vi "SparaRead.vi"(1 "Test Summary":string) -> (0 "判定结果":bool[](array[boolean]))   [LabVIEW 2011]
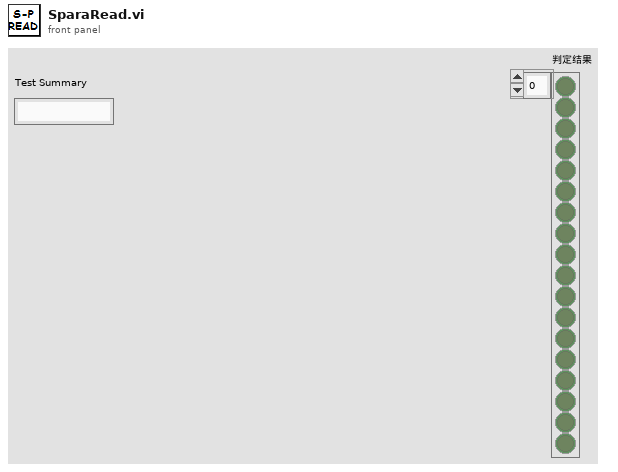
[diagram p1: front panel]
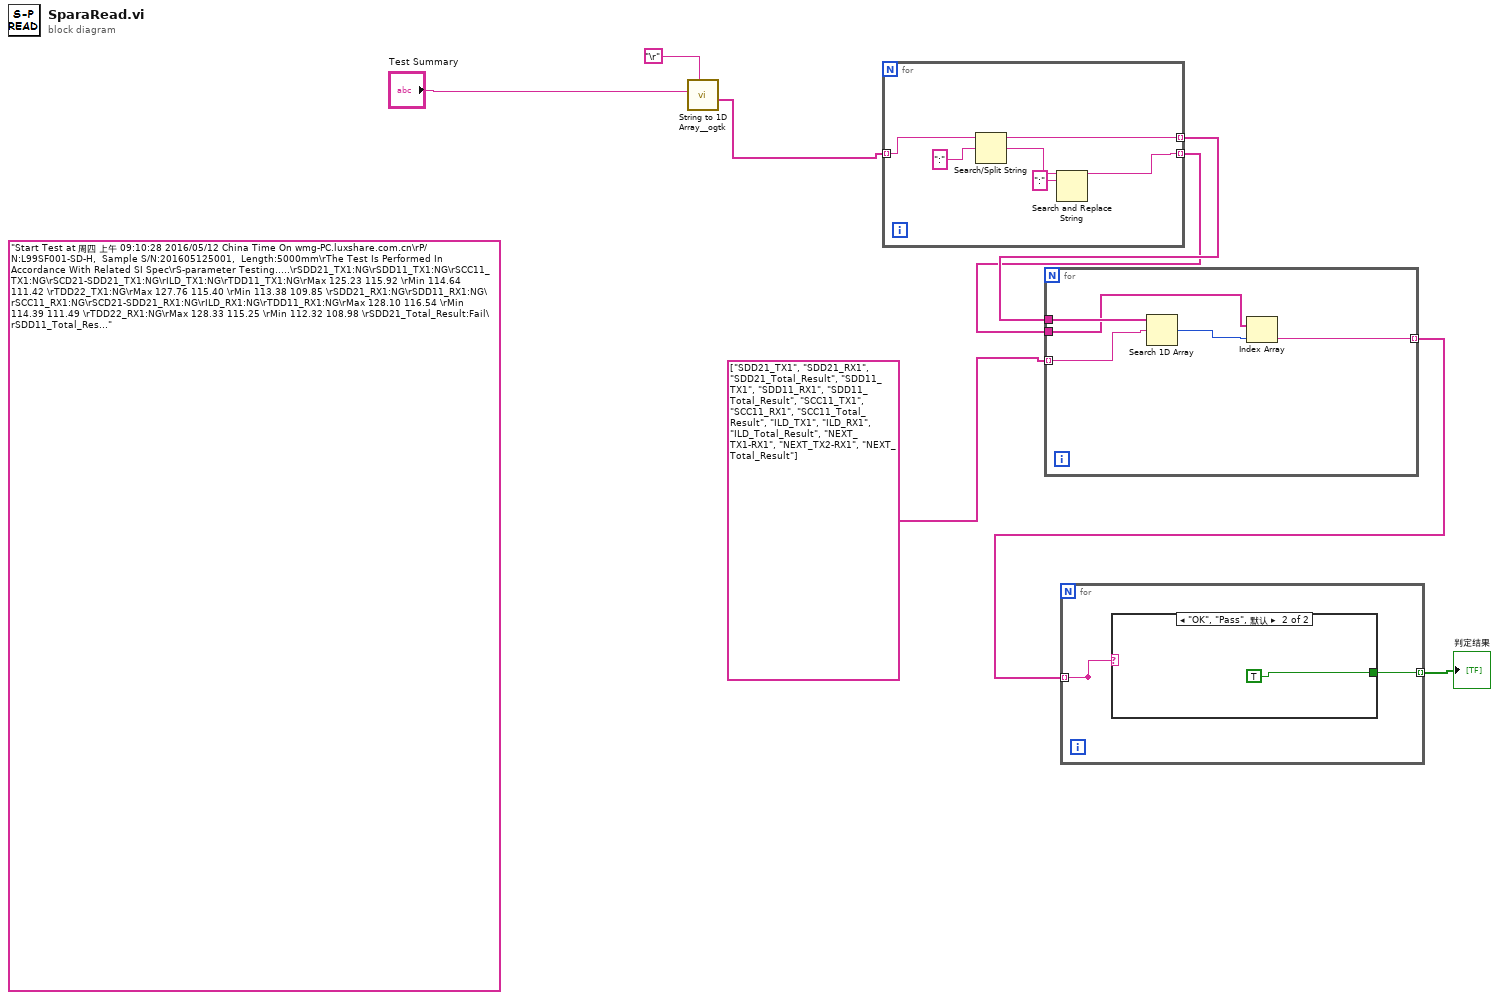
[diagram p0: block diagram]
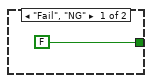
[diagram p2: hidden frame]
diagram:
  (unwired) "Start Test at 周四 上午 09:10:28 2016/05/12 China Time On wmg-PC.luxshare.com.cn\rP/N:L99SF001-SD-H,  Sample S/N:201605125001,  Length:5000mm\rThe Test Is Performed In Accordance With Related SI Spec\rS-parameter Testing.....\rSDD21_TX1:NG\rSDD11_TX1:NG\rSCC11_TX1:NG\rSCD21-SDD21_TX1:NG\rILD_TX1:NG\rTDD11_TX1:NG\rMax 125.23 115.92 \rMin 114.64 111.42 \rTDD22_TX1:NG\rMax 127.76 115.40 \rMin 113.38 109.85 \rSDD21_RX1:NG\rSDD11_RX1:NG\rSCC11_RX1:NG\rSCD21-SDD21_RX1:NG\rILD_RX1:NG\rTDD11_RX1:NG\rMax 128.10 116.54 \rMin 114.39 111.49 \rTDD22_RX1:NG\rMax 128.33 115.25 \rMin 112.32 108.98 \rSDD21_Total_Result:Fail\rSDD11_Total_Result:Fail\rSCC11_Total_Result:Fail\rSCD21-SDD21_Total_Result:Fail\rILD_Total_Result:Fail\rTDD11_Total_Result:Fail\rTDD22_Total_Result:Fail\rNEXT Testing.....\rNEXT_TX1-RX1:OK\rNEXT_TX2-RX1:OK\rNEXT_Total_Result:Pass\nWrite EEprom\nRead EEprom\nPort 0: FAIL\nPort 1: FAIL\nLabel has been printed!\n201605125001 :Test Finished !\rEnded Test At 周四 上午 09:11:18 2016/05/12 China Time.  Test Time: 49.969858s"
  n1 = call <userlib>:"String to 1D Array__ogtk.vi"("delimiter (Tab)"="\r", "string"="Test Summary") -> ("Array of Strings"=w6:string[])  [unwired: 9 in]
  n2 = for {
    tunnel: w6 -> [w14] mode=indexing
    tunnel: [w12] -> w5 mode=indexing
    tunnel: [w9] -> w4 mode=indexing
    n3 = Search/Split String(string=w14, search string/char (-)=":" ("搜索字符串/字符(-)")) -> (substring before match=w12:string, match + rest of string=w11:string)  [unwired: 1 in, 1 out]
    n4 = Search and Replace String(input string=w11, search string=":" ("搜索字符串")) -> (result string=w9:string)  [unwired: 6 in, 3 out]
  }
  n5 = for {
    tunnel: string[] ["SDD21_TX1", "SDD21_RX1", "SDD21_Total_Result", "SDD11_TX1", "SDD11_RX1", "SDD11_Total_Result", "SCC11_TX1", "SCC11_RX1", "SCC11_Total_Result", "ILD_TX1", "ILD_RX1", "ILD_Total_Result", "NEXT_TX1-RX1", "NEXT_TX2-RX1", "NEXT_Total_Result"] ("数组") -> [w19] mode=indexing
    tunnel: w5 -> [w18]
    tunnel: w4 -> [w17]
    tunnel: [w15] -> w2 mode=indexing
    n6 = Search 1D Array(1D array=w18, element=w19) -> (index of element=w16:i32)  [unwired: 1 in]
    n7 = Index Array(array=w17, index=w16) -> (element=w15:string)
  }
  n8 = for {
    tunnel: [w21] -> _ mode=indexing
    tunnel: w2 -> [w21] mode=indexing
    tunnel: [w20] -> w1 mode=indexing
    n9 = case shown="\"OK\", \"Pass\", 默认" w21 {
      tunnel: [FALSE TRUE] -> w20
      frame "Fail", "NG" {
      }
      frame "OK", "Pass", Default {
      }
    }
  }
  "判定结果" <- w1
